vi "Print VI FP as PDF File.vi"(6 "Report.File Path":path=path "E:/DRS Projects/FOD Reports/Report Test.pdf", 7 "VI path":path=path "E:/DRS Projects/FOD Detection/SubVIs/Save Report to PDF_Test.vi", 8 "error in (no error)":errorcluster) -> (0 "error out":errorcluster)   [LabVIEW 2020]
uses:
  <vilib>/printing/EasyPrintingControls.llb/contents.ctl
  <vilib>/Utility/NIReport.llb/Report Type (with Quick Print).ctl
  <vilib>/Utility/NIReport.llb/NI_report.lvclass
  <vilib>/Utility/NIReport.llb/NI_ReportGenerationCore.lvlib
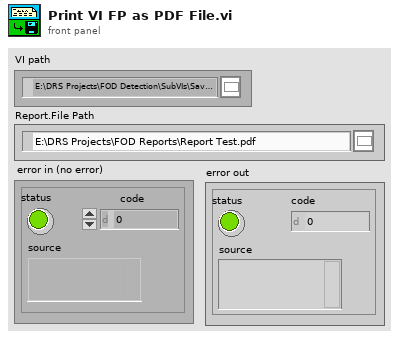
[diagram p1: front panel]
types:
  T1 = typedef "NI_ReportGenerationCore.lvlib/Report Type (with Quick Print).ctl" = enum16{"Quick Print", "HTML", "Word", "Excel"}
  T2 = typedef "NI_ReportGenerationCore.lvlib/contents.ctl" = u16
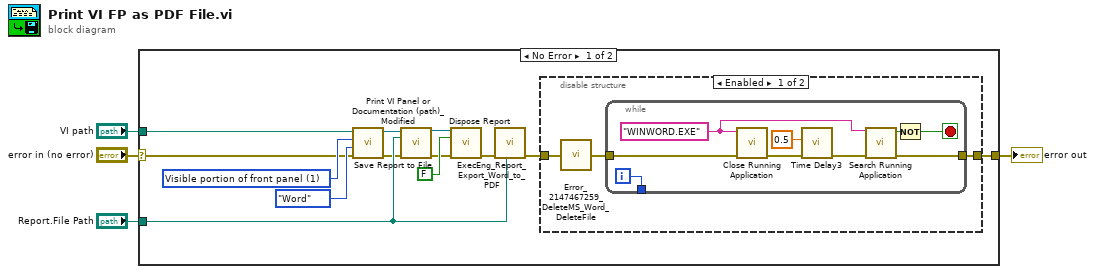
[diagram p0: block diagram]
diagram:
  n1 = case shown="No Error" "error in (no error)" {
    selector: "error in (no error)" -> [w12 w31]
    tunnel: "VI path" -> [w10 _]
    tunnel: [w6 w31] -> w3
    tunnel: "Report.File Path" -> [w13 _]
    frame No Error {
      w17 = T2 1 items=["Complete front panel", "Visible portion of front panel", "Icon, description, panel and diagram", "Documentation: Using the panel", "Documentation: Using as a subVI", "Documentation: Complete", "Documentation: Custom"] ("contents (complete front panel)")
      n2 = call "Print VI Panel or Documentation (path)_Modified.vi"("error in (no error)"=w12, "report type (Quick Print)"=Report_Type_(with_Quick_Print)."Word", "contents (complete front panel)"=w17, "VI path"=w10) -> ("error out"=w11:errorcluster, "report out"=w15:refnum<class "NI_report.lvclass">)  [unwired: 6 in]
      n3 = call-dynamic "Save Report to File.vi"("report in"=w15, "report file path"=w13, "error in (no error)"=w11) -> ("report out"=w14:refnum<class "NI_report.lvclass">, "error out"=w5:errorcluster)  [unwired: 11 in]
      n4 = call-dynamic "Dispose Report.vi"("report in"=w14, "wait until printing completed? (T)"=FALSE, "error in (no error)"=w5) -> ("error out"=w8:errorcluster)  [unwired: 12 in]
      n5 = call "ExecEng_Report_Export_Word_to_PDF.vi"("File path (docx)"=w13, "error in (no error)"=w8) -> ("error out"=w7:errorcluster)  [unwired: 8 in, 1 out]
      n6 = disable-structure shown="Enabled" {
        disable-tunnel: w7 -> [w20 w30]
        disable-tunnel: [w18 w30] -> w6
        frame Enabled {
          n7 = call "Error_2147467259_DeleteMS_Word_DeleteFile.vi"("error in"=w20) -> ("error out"=w19:errorcluster)  [unwired: 13 in, 1 out]
          n8 = while {
            tunnel: w19 -> [w29]
            tunnel: [w28] -> w18
            tunnel: [w21] -> _
            i -> [w21]
            stop <- w22 stop-if-true
            w27 = "WINWORD.EXE" ("App name")
            n9 = call "Close Running Application.vi"("Error In"=w29, "App name"=w27) -> ("Error Out"=w26:errorcluster)  [unwired: 8 in, 1 out]
            n10 = call "Time Delay3"("error in (no error)"=w26, "Delay Time (s)"=0.5) -> ("error out"=w25:errorcluster)  [unwired: 9 in]
            n11 = call "Search Running Application.vi"("Error In"=w25, "App name"=w27) -> ("Error Out"=w28:errorcluster, "Searched App is running"=w23:bool)  [unwired: 8 in]
            n12 = Not(x=w23) -> (.not. x?=w22:bool)
          }
        }
        frame Disabled {
        }
      }
    }
    frame Error {
    }
  }
  "error out" <- w3
